vi "OpticalLobe.vi"() -> (1 "Working Image":T1(plugin-control), 2 "Occupancy Grid":T1(plugin-control))   [LabVIEW 2011]
uses:
  WhereAmI.ctl
  <vilib>/userdefined/High Color/IMAQdx.ctl
  <vilib>/vision/Image Controls.llb/IMAQ Image.ctl
  Position.ctl
  OccGrid.ctl
  <vilib>/vision/driver/NI_Vision_Acquisition_Software.lvlib
panel:
  out "x":sgl[](array[numeric])
  out "y":sgl[](array[numeric])
  out "OccupancyGrid (Raw Data)":i8[][](array[numeric])
  out "Working":bool
  in  "Camera/File?":bool
  in  "Camera Name":T2
  in  "Image file name":string="real pool targets rotated.bmp"
  out "Dock":cluster{"x":sgl, "y":sgl}
  out "Bouy 1":cluster{"x":sgl, "y":sgl}
  out "Boat":T3
  out "Nothing":cluster{"x":sgl, "y":sgl}
  in  "stop":bool
  out "error out":errorcluster
  # "File"
  # "Camera"
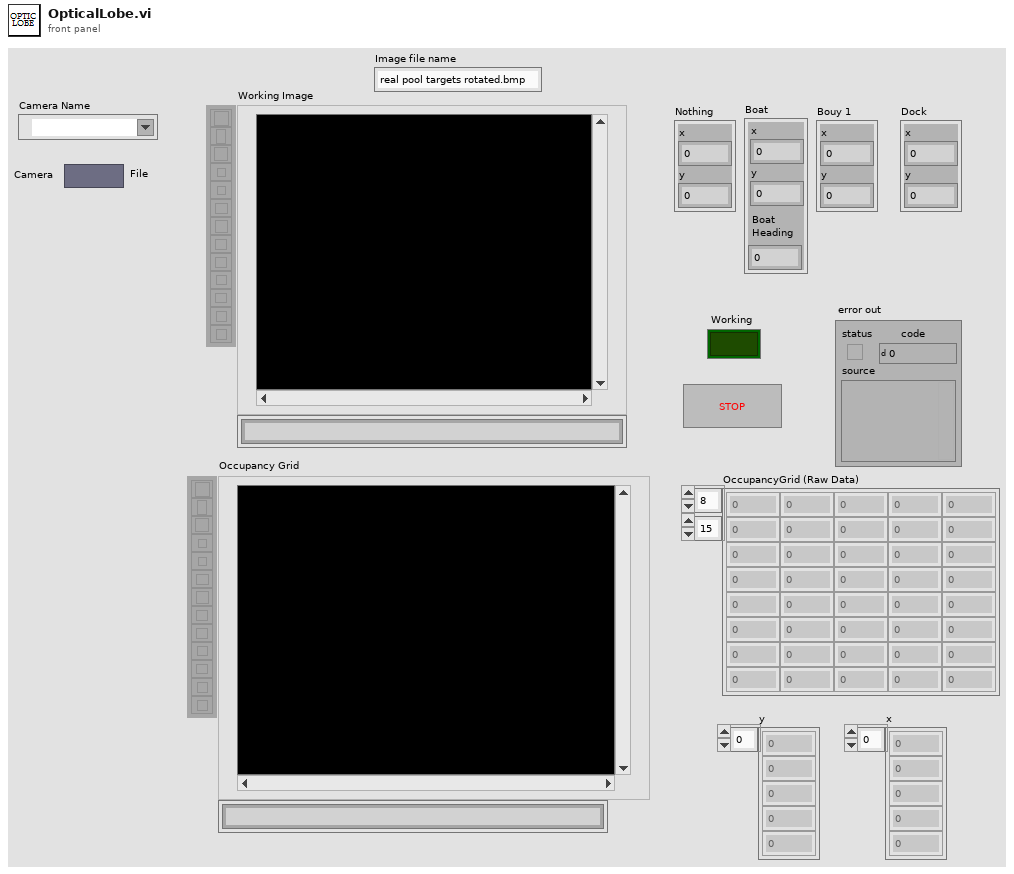
[diagram p1: front panel]
types:
  T1 = typedef "IMAQ Image.ctl" = refnum<image>
  T2 = typedef "IMAQdx.ctl" = refnum<k21>
  T3 = typedef "WhereAmI.ctl" = cluster{"x":sgl, "y":sgl, "Boat\nHeading":sgl}
  T4 = typedef "Image Type" = u32
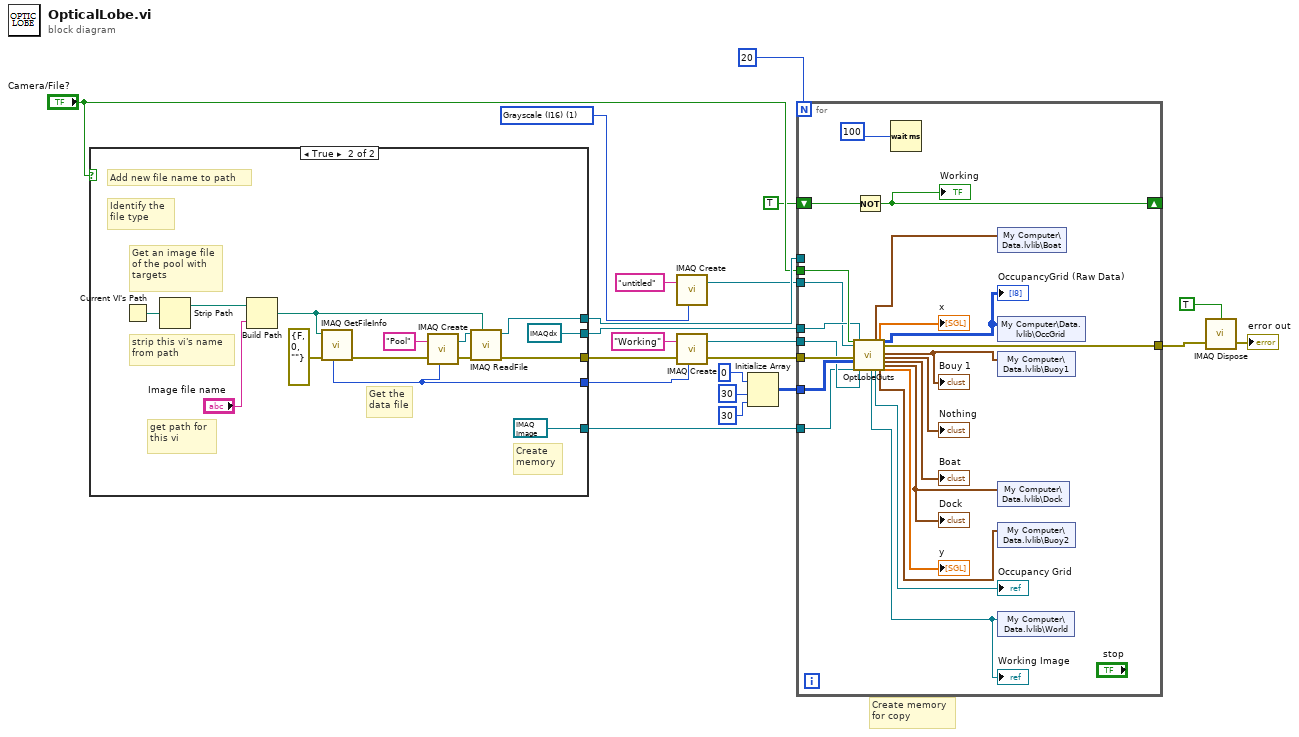
[diagram p0: block diagram]
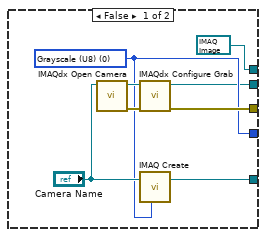
[diagram p2: hidden frame]
diagram:
  w5 = T4 1 items=["Grayscale (U8)", "Grayscale (I16)", "Grayscale (SGL)", "Complex (CSG)", "RGB (U32)", "HSL (U32)", "RGB (U64)", "Grayscale (U16)"] ("Image Type")
  # "Create memory\nfor copy"
  n1 = case shown="True" "Camera/File?" {
    tunnel: [T1 refnum ("Image Out") w34] -> w13
    tunnel: [w26 w33] -> w18
    tunnel: [w25 w32] -> w17
    tunnel: [w24 T1 refnum ("New Image")] -> w15
    tunnel: [w23 T2 refnum ("Session Out")] -> w14
    frame False {
      w25 = T4 0 items=["Grayscale (U8)", "Grayscale (I16)", "Grayscale (SGL)", "Complex (CSG)", "RGB (U32)", "HSL (U32)", "RGB (U64)", "Grayscale (U16)"] ("Image Type")
      n2 = call <vilib>:"IMAQdx Open Camera.vi"("Session In"="Camera Name") -> ("error out"=w29:errorcluster, "Session Out"=w28:T2)  [unwired: 2 in, 7 out]
      n3 = call <vilib>:"IMAQdx Configure Grab.vi"("error in"=w29, "Session In"=w28) -> ("error out"=w26:errorcluster, "Session Out"=w23:T2)  [unwired: 8 out]
      n4 = call "IMAQ Create"("Image Name"="Camera Name", "Image Type"=w25) -> ("New Image"=w24:T1)  [unwired: 2 in, 2 out]
    }
    frame True {
      # "Add new file name to path"
      # "strip this vi's name \nfrom path"
      # "get path for \nthis vi"
      # "Get the \ndata file"
      # "Create \nmemory"
      # "Identify the \nfile type"
      # "Get an image file\nof the pool with\ntargets"
      n5 = Current VI's Path() -> (path=w37:path)
      n6 = Strip Path(path=w37) -> (stripped path=w36:path)  [unwired: 1 out]
      n7 = Build Path(base path=w36, name or relative path="Image file name") -> (appended path=w35:path)
      n8 = call "IMAQ GetFileInfo"("error in (no error)"=errorcluster {"status"=FALSE, "code"=0, "source"=""}, "File Path"=w35) -> ("error out"=w43:errorcluster, "Image Type"=w32:T4)  [unwired: 3 in, 5 out]
      n9 = call "IMAQ Create"("Image Name"="Pool", "Image Type"=w32, "error in (no error)"=w43) -> ("New Image"=w41:T1, "error out"=w39:errorcluster)  [unwired: 2 in]
      n10 = call "IMAQ ReadFile"("File Path"=w35, "error in (no error)"=w39, "Image"=w41) -> ("error out"=w33:errorcluster, "Image Out"=w34:T1)  [unwired: 4 in, 3 out]
    }
  }
  n11 = call "IMAQ Create"("Image Name"="untitled", "Image Type"=w5) -> ("New Image"=w6:T1)  [unwired: 3 in, 1 out]
  n12 = call "IMAQ Create"("Image Name"="Working", "Image Type"=w17, "error in (no error)"=w18) -> ("New Image"=w19:T1, "error out"=w21:errorcluster)  [unwired: 2 in]
  n13 = Initialize Array(i16 0 ("element"), 30 ("dimension size"), 30 ("dimension size")) -> (w7:i16[][])
  n14 = for {
    N: 20 ("Numeric") -> [_]
    tunnel: w21 -> [w60]
    tunnel: w19 -> [w45]
    tunnel: [w57] -> w3
    tunnel: w15 -> [w44]
    tunnel: w14 -> [w59]
    tunnel: w13 -> [_]
    tunnel: "Camera/File?" -> [w62]
    shift-right: [w63] -> _
    shift-left: TRUE -> [w64]
    tunnel: w7 -> [w61]
    tunnel: w6 -> [w48]
    n15 = call "OptLobeGuts.vi"("Boolean"=w62, "source"=w48, "error in (no error)"=w60, "Array"=w61, "New Image"=w44, "Session Out"=w59, "Image Dst"=w45) -> ("Working Image"=w55:T1, 16:"Boat"=w56:T3, "Occupancy Grid"=→"Occupancy Grid":T1, "x"=→"x":sgl[], "Buoy 2"=w47:cluster{"x":sgl, "y":sgl}, "OccupancyGrid (Raw Data)"=w46:i8[][], "error out"=w57:errorcluster, "Bouy 1"=w49:cluster{"x":sgl, "y":sgl}, "Nothing"=→"Nothing":cluster{"x":sgl, "y":sgl}, 25:"Boat"=→"Boat":T3, "Dock"=w50:cluster{"x":sgl, "y":sgl}, "y"=→"y":sgl[])  [unwired: 8 in, 1 out]
    "Working Image" <- w55
    "Bouy 1" <- w49
    "Dock" <- w50
    "OccupancyGrid (Raw Data)" <- w46
    n16 = Not(x=w64) -> (.not. x?=w63:bool)
    "Working" <- w63
    n17 = Wait (ms)(milliseconds to wait=u32 100) -> ()  [unwired: 1 out]
    n18 = shared-variable "My Computer\\Data.lvlib\\Boat"(w56) -> ()  [unwired: 1 in, 1 out]
    n19 = shared-variable "My Computer\\Data.lvlib\\OccGrid"(w46) -> ()  [unwired: 1 in, 1 out]
    n20 = shared-variable "My Computer\\Data.lvlib\\Buoy1"(w49) -> ()  [unwired: 1 in, 1 out]
    n21 = shared-variable "My Computer\\Data.lvlib\\Dock"(w50) -> ()  [unwired: 1 in, 1 out]
    n22 = shared-variable "My Computer\\Data.lvlib\\Buoy2"(w47) -> ()  [unwired: 1 in, 1 out]
    n23 = shared-variable "My Computer\\Data.lvlib\\World"(w55) -> ()  [unwired: 1 in, 1 out]
  }
  n24 = call "IMAQ Dispose"("All Images? (No)"=TRUE, "error in (no error)"=w3) -> ("error out"=→"error out":errorcluster)  [unwired: 4 in]
